vi "AddDataProcessor.vi"(0 "Microscope in":refnum<class "Microscope.lvclass">, 5 "Label":string, 7 "DataProcessor":refnum<class "DataProcessor.lvclass">, 9 "RegisterInPipleline?(F)":bool=TRUE, 11 "error in (no error)":errorcluster) -> (4 "Microscope out":refnum<class "Microscope.lvclass">, 15 "error out":errorcluster)   [LabVIEW 2020, in "Microscope.lvlib" / "Microscope.lvclass"]
uses:
  Microscope.lvclass
  C:/Program Files/National Instruments/LabVIEW 2020/vi.lib/ActorFramework/Actor/Actor.lvclass
  Logic Layer/DataProcessor/DataProcessor/DataProcessor.lvclass
  <vilib>/ActorFramework/Message Enqueuer/Message Enqueuer.lvclass
  <vilib>/ActorFramework/Actor/Actor.lvclass
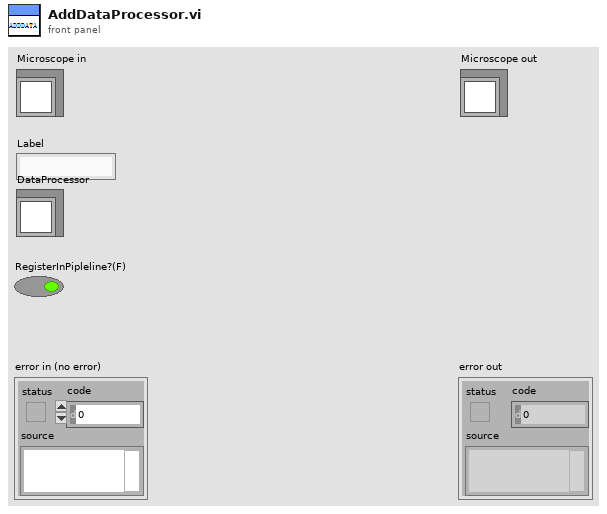
[diagram p1: front panel]
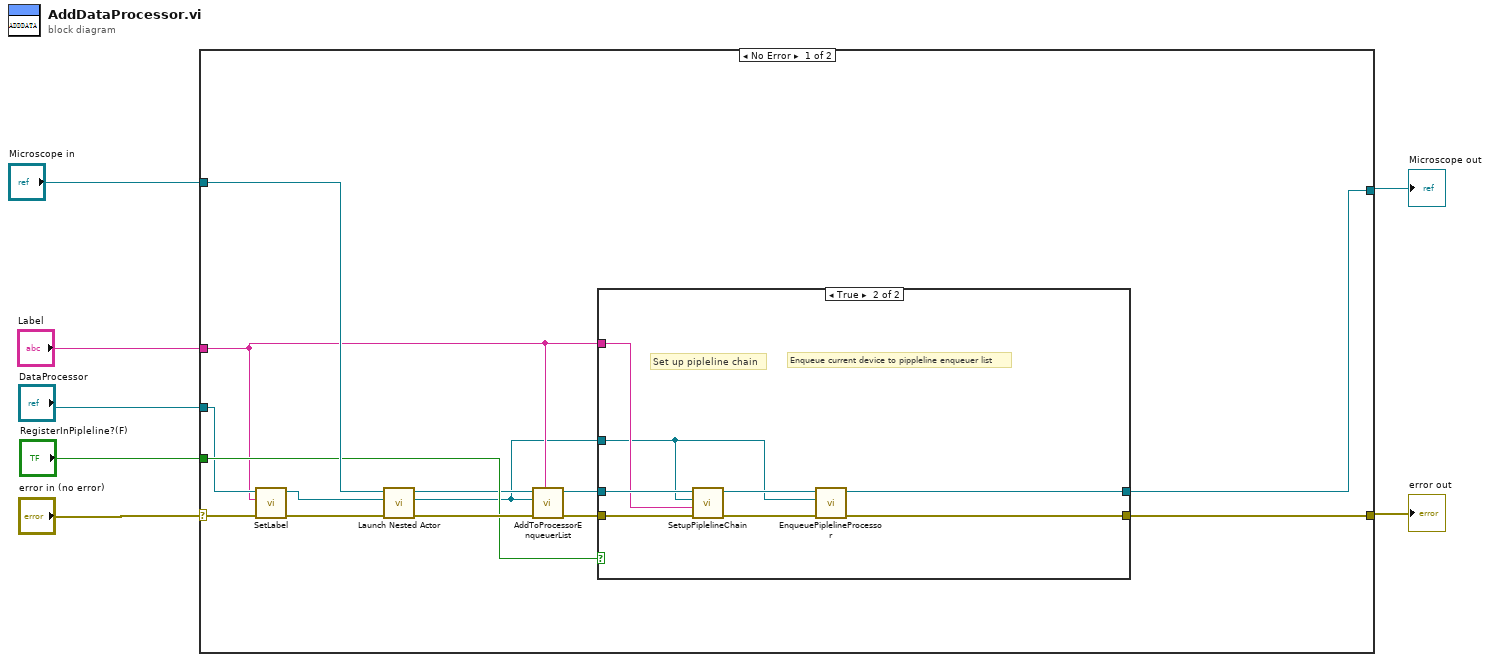
[diagram p0: block diagram]
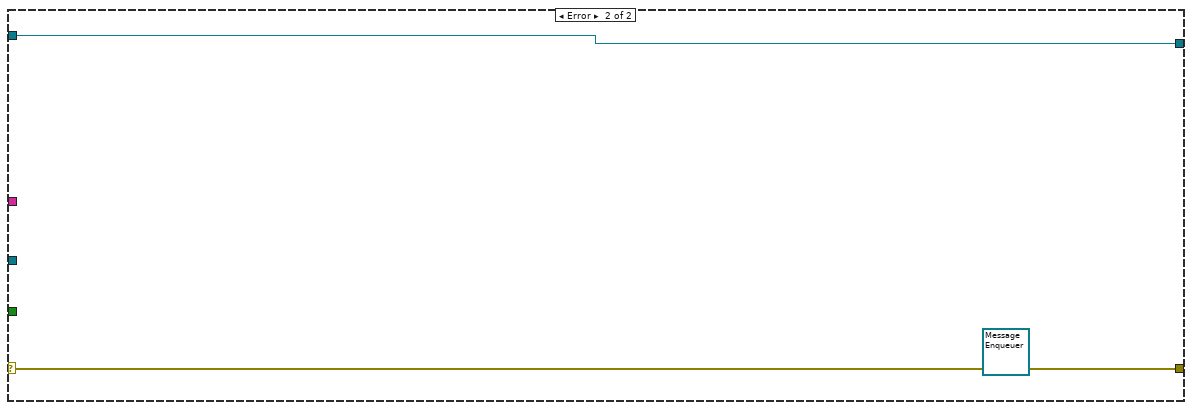
[diagram p3: hidden frame]
diagram:
  n1 = case shown="No Error" "error in (no error)" {
    selector: "error in (no error)" -> [w21 w33]
    tunnel: [w8 w33] -> w6
    tunnel: [w17 w32] -> w4
    tunnel: "Microscope in" -> [w19 w32]
    tunnel: "DataProcessor" -> [w15 _]
    tunnel: "Label" -> [w11 _]
    tunnel: "RegisterInPipleline?(F)" -> [w18 _]
    frame No Error {
      n2 = call-dynamic "SetLabel.vi"("error in (no error)"=w21, "Label"=w11, "DataProcessor in"=w15) -> ("error out"=w16:errorcluster, "DataProcessor out"=w14:refnum<class "DataProcessor.lvclass">)  [unwired: 7 in]
      n3 = call <vilib>:"Launch Nested Actor.vi"("error in (no error)"=w16, "Nested Actor"=w14, "Caller Actor in"=w19) -> ("error out"=w20:errorcluster, "Nested Actor's Enqueuer"=w9:refnum<class "Message Enqueuer.lvclass">, "Caller Actor out"=w13:refnum<class "Microscope.lvclass">)  [unwired: 6 in]
      n4 = call-dynamic "AddToProcessorEnqueuerList.vi"("error in (no error)"=w20, "Label"=w11, "ProcessorEnqueuer"=w9, "Microscope in"=w13) -> ("error out"=w10:errorcluster, "Microscope out"=w12:refnum<class "Microscope.lvclass">)  [unwired: 4 in, 2 out]
      n5 = case shown="True" w18 {
        tunnel: w12 -> [w23 w31]
        tunnel: [w23 w26] -> w17
        tunnel: w11 -> [_ w25]
        tunnel: w10 -> [w22 w30]
        tunnel: w9 -> [_ w24]
        tunnel: [w22 w28] -> w8
        frame False {
        }
        frame True {
          # "Enqueue current device to pippleline enqueuer list"
          # "Set up pipleline chain"
          n6 = call-dynamic "SetupPiplelineChain.vi"("error in (no error)"=w30, "Destination"=w25, "Enqueuer"=w24, "Microscope in"=w31) -> ("error out"=w29:errorcluster, "Microscope out"=w27:refnum<class "Microscope.lvclass">)  [unwired: 6 in]
          n7 = call-dynamic "EnqueuePiplelineProcessor.vi"("error in (no error)"=w29, "DeviceEnqueuer"=w24, "Microscope in"=w27) -> ("error out"=w28:errorcluster, "Microscope out"=w26:refnum<class "Microscope.lvclass">)  [unwired: 7 in]
        }
      }
    }
    frame Error {
      (unwired) refnum<class "Message Enqueuer.lvclass"> refnum ("Nested Actor's Enqueuer")
    }
  }
  "error out" <- w6
  "Microscope out" <- w4
